vi "Main - Output Wavedorm to drive Galvo.vi"(11 "Element address final":u32) -> (3 "Waveform Output Done":bool)   [LabVIEW 2015]
uses:
  <vilib>/Platform/TimedLoop/XDataNode/timing_clust.ctl
  <vilib>/Platform/TimedLoop/XDataNode/nitl_modes.ctl
  <vilib>/Platform/TimedLoop/XDataNode/wakeup.ctl
  DRAM data index.ctl
  <vilib>/rvi/Emulation/niFpgaGetClockAttributes.vi
  <vilib>/rvi/Emulation/niFpgaSctlEmulationGetInTimedLoop.vi
  <vilib>/rvi/Emulation/niFpgaEmulationReportErrorSimple.vi
  <vilib>/rvi/eio/common/nirviEmuTemplateMethod_errors.vi
  <vilib>/rvi/Emulation/niFpgaCriticalErrorInLSC.vi
  <vilib>/eio/EIONode/EIONode.xnode
  <vilib>/Platform/TimedLoop/XDataNode/XDataNode.xnode
  <vilib>/Platform/TimedLoop/XDataNode/XDNodeRunTimeDep.lvlib
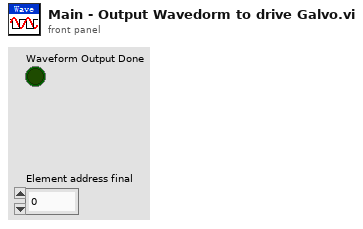
[diagram p1: front panel]
types:
  T1 = enum16{"Nodes setting", "Waveform Generation", "Stop"}
  T2 = typedef "XDNodeRunTimeDep.lvlib/timing_clust.ctl" = cluster{"Expected End [f-1]":u64, "Actual End [f-1]":u64, "Finished Late? [f-1]":bool, "Expected End [i-1]":u64, "Actual End [i-1]":u64, "Finished Late? [i-1]":bool, "Expected Start [i]":u64, "Actual Start [i]":u64, "Expected Start [f]":u64, "Actual Start [f]":u64, "Source Name":string, "Structure Name":string, "Period":i64, "Deadline":i64, "Offset":i64, "Start":i64, "Priority":i32, "Timeout":i32, "Mode":T3, "Wakeup Reason":T4, "Error":errorcluster, "Source Type":string, "Secondary Source Type":string, "Global End Time":u64, "Global Start Time":u64, "Frame Duration":u64, "Iteration Duration":u64, "Assigned CPU":i32, "I/O Scan Engine Mode":u32}
  T3 = typedef "XDNodeRunTimeDep.lvlib/nitl_modes.ctl" = enum32{"No Change", "Process missed periods, maintain original phase", "Discard missed periods, maintain original phase", "Process missed periods, ignore original phase", "Discard missed periods, ignore original phase"}
  T4 = typedef "XDNodeRunTimeDep.lvlib/wakeup.ctl" = enum32{"Normal", "Aborted", "Asynchronous wakeup", "Timing source error", "Timed loop error", "Timeout"}
  T5 = typedef "DRAM data index.ctl" = enum16{"Numeric 1", "Numeric 2", "Numeric 3", "Numeric 4", "Numeric 5", "Numeric 6", "Numeric 7", "Numeric 8", "Numeric 9", "Numeric 10", "Numeric 11", "Numeric 12", "Numeric 13", "Numeric 14", "Numeric 15", "Numeric 16"}
  T6 = cluster{"Numeric 1":u32, "Numeric 2":u32, "Numeric 3":u32, "Numeric 4":u32, "Numeric 5":u32, "Numeric 6":u32, "Numeric 7":u32, "Numeric 8":u32, "Numeric 9":u32, "Numeric 10":u32, "Numeric 11":u32, "Numeric 12":u32, "Numeric 13":u32, "Numeric 14":u32, "Numeric 15":u32, "Numeric 16":u32}
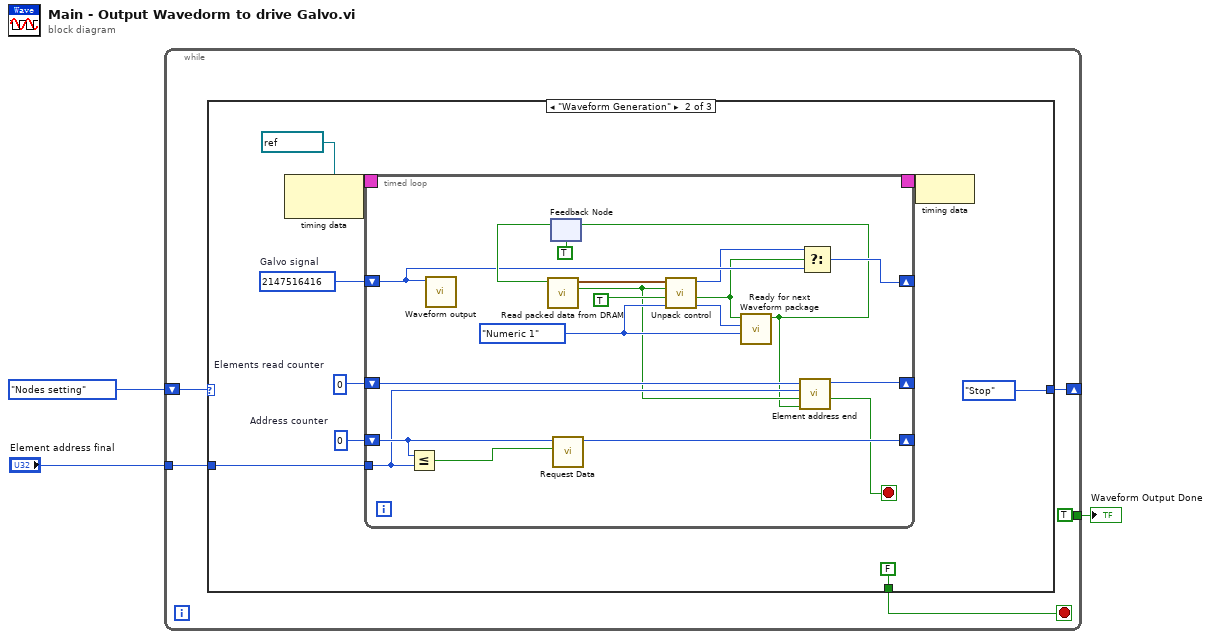
[diagram p0: block diagram]
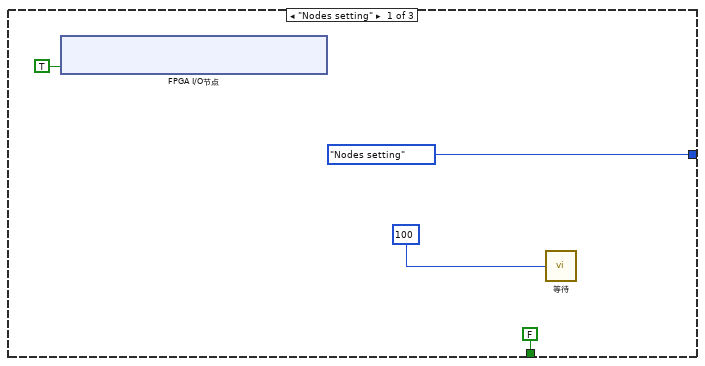
[diagram p2: hidden frame]
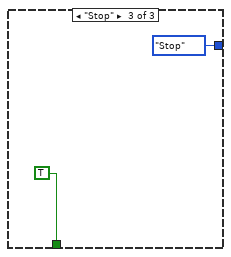
[diagram p3: hidden frame]
diagram:
  n1 = while {
    shift-right: [w7] -> _
    shift-left: T1."Nodes setting" -> [w8]
    tunnel: "Element address final" -> [w6]
    tunnel: [TRUE] -> w1
    stop <- w5 stop-if-true
    n2 = case shown="\"Waveform Generation\"" w8 {
      tunnel: [T1."Nodes setting" T1."Stop" T1."Stop"] -> w7
      tunnel: w6 -> [_ w16 _]
      tunnel: [FALSE FALSE TRUE] -> w5
      frame "Nodes setting" {
        n3 = xnode "FPGA I/O节点"("IO Module\\Shutter(DDCA_PFI1_WRITE)"=TRUE ("IO Module\\Shutter(DDCA_PFI1_WRITE)")) -> ()  [unwired: 1 in, 1 out]
        n4 = call "等待"("Count(mSec)"=u32 100) -> ()  [unwired: 1 out]
      }
      frame "Waveform Generation" {
        w13 = u32 0  # Elements read counter
        w17 = u32 0  # Address counter
        w18 = u32 2147516416  # Galvo signal
        n5 = node-c288(refnum<k21> "5MHz" ("源名称")) -> (w21:T2)
        n6 = timed-loop {
          timing: w21 -> [_]
          timing-out: [_] -> w20
          shift-right: [w29] -> _
          shift-left: w18 -> [w31]
          tunnel: w16 -> [w26]
          shift-right: [w33] -> _
          shift-left: w17 -> [w34]
          shift-right: [w25] -> _
          shift-left: w13 -> [w27]
          stop <- w24 stop-if-true
          w37 = DRAM_data_index."Numeric 1" ("DRAM pack index out")
          n7 = Less Or Equal?(x=w34, y=w26) -> (x <= y?=w32:bool)
          n8 = call "Waveform output.vi"("Galvo signal"=w31) -> ()  [unwired: 11 in]
          n9 = feedback #1(TRUE) -> (w36:bool)
          n10 = call "Read packed data from DRAM.vi"("Output ready"=w36) -> ("Output Valid§"=w23:bool, "Data"=w40:T6)  [unwired: 9 in]
          n11 = call "Request Data.vi"("Elements remain?"=w32, "Address counter"=w34) -> ("Address counter output"=w33:u32)  [unwired: 9 in]
          n12 = call "Unpack control.vi"("DRAM pack index init"=w37, "enable unpack"=TRUE, "input valid"=w23, "Data"=w40) -> ("DRAM pack index out"=w38:T5, "output valid?"=w28:bool, "Unpacked data"=w30:u32)  [unwired: 5 in]
          n13 = call "Ready for next Waveform package.vi"("DRAM pack index in"=w37, "DRAM pack index out"=w38, "output valid?"=w28) -> ("Ready for next package"=w22:bool)  [unwired: 8 in]
          n14 = feedback-in #1(w22) -> ()
          n15 = call "Element address end.vi"("Last package unpacked"=w22, "Output Valid"=w23, "Element address final"=w26, "Elements read counter"=w27) -> ("All elements read"=w24:bool, "Next element address"=w25:u32)  [unwired: 6 in]
          n16 = Select(t=w30, s=w28, f=w31) -> (s? t:f=w29:u32)
        }
        n17 = node-c288(w20) -> ()
      }
      frame "Stop" {
      }
    }
  }
  "Waveform Output Done" <- w1
